vi "generate_list.vi"(0 "Upper bound":dbl, 7 "Step Size":dbl, 11 "Lower Bound":dbl) -> (8 "Array":dbl[](array[numeric]))   [LabVIEW 2023]
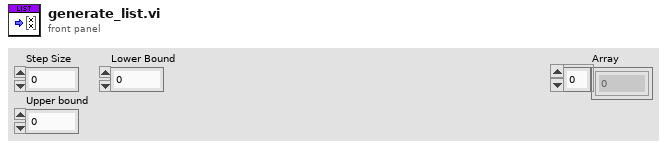
[diagram p1: front panel]
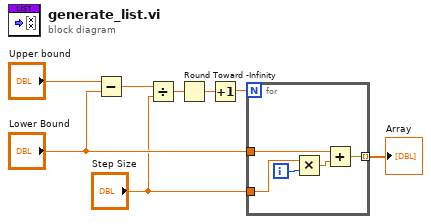
[diagram p0: block diagram]
diagram:
  n1 = Subtract(x="Upper bound", y="Lower Bound") -> (x-y=w5:dbl)
  n2 = Divide(x=w5, y="Step Size") -> (x/y=w6:dbl)
  n3 = Round Toward -Infinity(1:w6) -> (0:w7:dbl)
  n4 = Increment(x=w7) -> (x+1=w8:dbl)
  n5 = for {
    N: w8 -> [_]
    tunnel: "Lower Bound" -> [w12]
    tunnel: "Step Size" -> [w11]
    tunnel: [w9] -> w1 mode=indexing
    i -> [w10]
    n6 = Multiply(x=w11, y=w10) -> (x*y=w13:dbl)
    n7 = Add(x=w12, y=w13) -> (x+y=w9:dbl)
  }
  "Array" <- w1
